vi "Project Initializer.vi"(8 "error in (no error)":errorcluster, 10 "New Project Name":string="MyNiceProject", 11 "Template Source .lvproj":path) -> ()   [LabVIEW 2022 SP3]
panel:
  out "error out":errorcluster
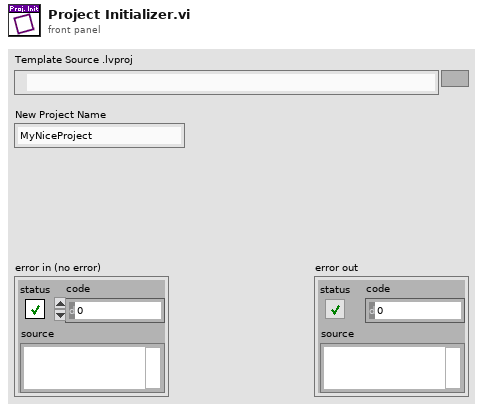
[diagram p1: front panel]
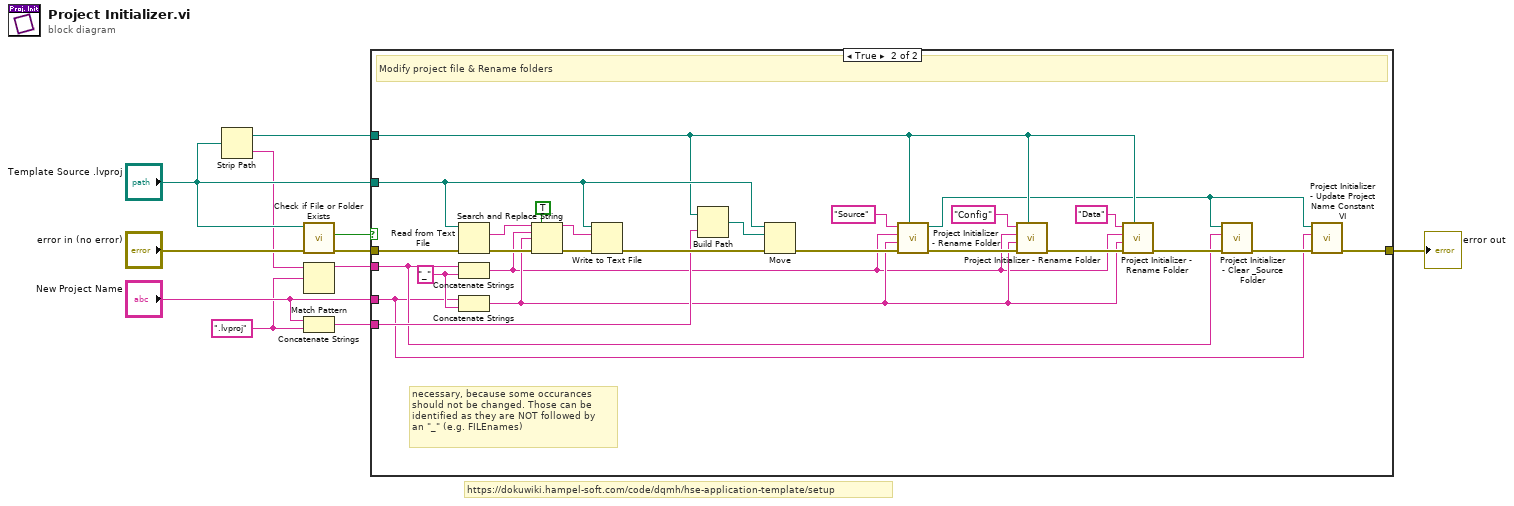
[diagram p0: block diagram]
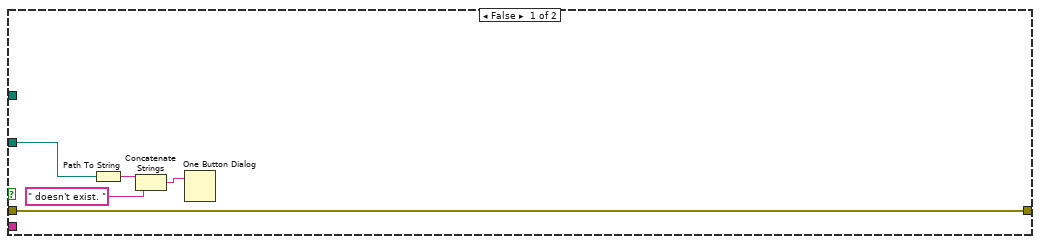
[diagram p2: hidden frame]
diagram:
  w3 = ".lvproj" ("string")
  # "https://dokuwiki.hampel-soft.com/code/dqmh/hse-application-template/setup"
  n1 = Strip Path(path="Template Source .lvproj") -> (stripped path=w8:path, name=w1:string)
  n2 = call <vilib>:"Check if File or Folder Exists.vi"("error in (no error)"="error in (no error)", "path"="Template Source .lvproj") -> ("error out"=w10:errorcluster, "file or folder exists?"=w11:bool)  [unwired: 7 in, 1 out]
  n3 = Match Pattern(string=w1, regular expression=w3) -> (before substring=w2:string)  [unwired: 1 in, 3 out]
  n4 = Concatenate Strings("New Project Name", w3) -> (w7:string)
  n5 = case shown="True" w11 {
    tunnel: "Template Source .lvproj" -> [w16 w24]
    tunnel: w10 -> [w12 w41]
    tunnel: w2 -> [_ w20]
    tunnel: "New Project Name" -> [_ w17]
    tunnel: [w12 w19] -> w5
    tunnel: w8 -> [_ w21]
    tunnel: w7 -> [_ w33]
    frame False {
      n6 = Path To String(path=w16) -> (string=w15:string)
      n7 = Concatenate Strings(w15, " doesn't exist. " ("string")) -> (w14:string)
      n8 = One Button Dialog(message=w14) -> ()  [unwired: 1 in, 1 out]
    }
    frame True {
      w38 = "_" ("string")
      # "necessary, because some occurances \nshould not be changed. Those can be \nidentified as they are NOT followed by \nan \"_\" (e.g. FILEnames)"
      # "Modify project file & Rename folders"
      n9 = Read from Text File(file (use dialog)=w24, error in=w41) -> (text=w40:string, error out=w42:errorcluster)  [unwired: 2 in, 2 out]
      n10 = Concatenate Strings(w20, w38) -> (w25:string)
      n11 = Concatenate Strings(w17, w38) -> (w29:string)
      n12 = Search and Replace String(replace all?=TRUE ("replace all? (F)"), input string=w40, search string=w25, replace string=w29, error in=w42) -> (result string=w36:string, error out=w37:errorcluster)  [unwired: 3 in, 2 out]
      n13 = Write to Text File(file (use dialog)=w24, text=w36, error in=w37) -> (error out=w35:errorcluster)  [unwired: 1 in, 2 out]
      n14 = Build Path(base path=w21, name or relative path=w33) -> (appended path=w34:path)
      n15 = Move(source path=w24, error in=w35, 10:w34) -> (error out=w32:errorcluster)  [unwired: 2 in, 2 out]
      n16 = call "Project Initializer - Rename Folder.vi"("Project Path"=w21, "error in (no error)"=w32, "Target Project Name"=w29, "Source Project Name"=w25, "Folder Suffix"="Source") -> ("error out"=w31:errorcluster, "New Folder Path"=w18:path)  [unwired: 5 in]
      n17 = call "Project Initializer - Rename Folder.vi"("Project Path"=w21, "error in (no error)"=w31, "Target Project Name"=w29, "Source Project Name"=w25, "Folder Suffix"="Config") -> ("error out"=w30:errorcluster)  [unwired: 5 in, 1 out]
      n18 = call "Project Initializer - Rename Folder.vi"("Project Path"=w21, "error in (no error)"=w30, "Target Project Name"=w29, "Source Project Name"=w25, "Folder Suffix"="Data") -> ("error out"=w23:errorcluster)  [unwired: 5 in, 1 out]
      n19 = call "Project Initializer - Clear _Source Folder.vi"("error in (no error)"=w23, "Source Project Name"=w20, "Project _Source Directory"=w18) -> ("error out"=w22:errorcluster)  [unwired: 8 in]
      n20 = call "Project Initializer - Update Project Name Constant VI.vi"("error in (no error)"=w22, "New Project Name"=w17, "New Project _Source Directory"=w18) -> ("error out"=w19:errorcluster)  [unwired: 8 in]
    }
  }
  "error out" <- w5
